vi "DB - [Config].[Controller].vi"(4 "[SystemId]":string="SRSB-A1", 6 "[PlantId]":string="4070", 7 "DB Connection":T2={"Open"=TRUE, "Close"=TRUE}, 8 "error in (no error)":errorcluster, 9 "DB.Schema.Table \nSRTRS.Config.Controller":string="SRTRS.Config.Controller", 10 "DB.Schema.Table\nSRTRS.Config.SysControlRelation":string="SRTRS.Config.SysControlRelation", 11 "connection reference":T1) -> (0 "SUMMARY":errorcluster, 2 "data":string[](array[string]), 3 "connection reference":T1)   [LabVIEW 2013]
uses:
  <vilib>/addons/database/Connection.llb/Conn ObjectReference.ctl
  Controls/DB - OpenClose.ctl
  <vilib>/addons/database/Connection.llb/Conn Execute.vi
  <vilib>/addons/database/Recordset.llb/Rec Fetch Recordset Data (R).vi
  <vilib>/addons/database/Recordset.llb/Rec Destroy - Connection.vi
  Controls/Global SRTRS.vi
  <vilib>/addons/database/Connection.llb/DB Tools Open Connec (String).vi
  <vilib>/addons/database/_DB Variant To Data/Database Variant To Data.xnode
  <vilib>/addons/database/NI_Database_API.lvlib
panel:
  out "Close":errorcluster
  in  "DB.Schema.Table \nNA":string
  out "SQL Statement":string
  out "Connection Information":T3={"Connection "="SQL Server 32bit HPEnvy", "Username"="admin", "Password"="admin123"}
  # "2014-10-27 14:11\n[IpAddress]                                                              [ChannelMapping]"
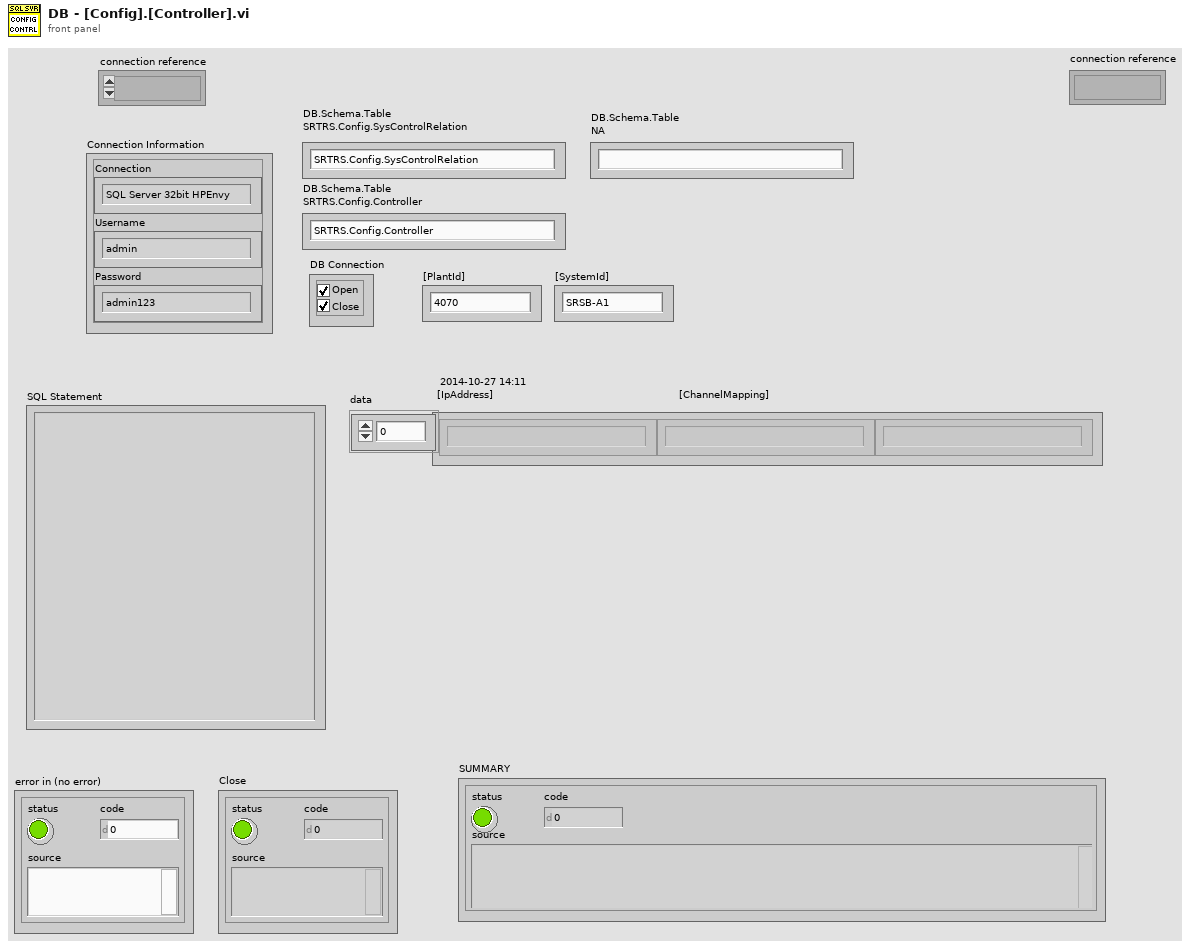
[diagram p1: front panel]
types:
  T1 = typedef "NI_Database_API.lvlib/Conn ObjectReference.ctl" = refnum<k1>
  T2 = typedef "DB - OpenClose.ctl" = cluster{"Open":bool, "Close":bool}
  T3 = cluster{"Connection ":string, "Username":string, "Password":string}
  T4 = typedef "Enum - InteractiveMode-SubVIMode.ctl" = enum16{"Interactive", "subVI Mode"}
  T5 = typedef "DB - DB.Schema.Table.ctl" = cluster{"DB":string, "Schema":string, "Table":string}
  T6 = typedef "Connection Information Cluster.ctl" = cluster{"Connection ":string, "Username":string, "Password":string}
  T7 = typedef "NI_Database_API.lvlib/Rec ObjectReference.ctl" = refnum<k1>
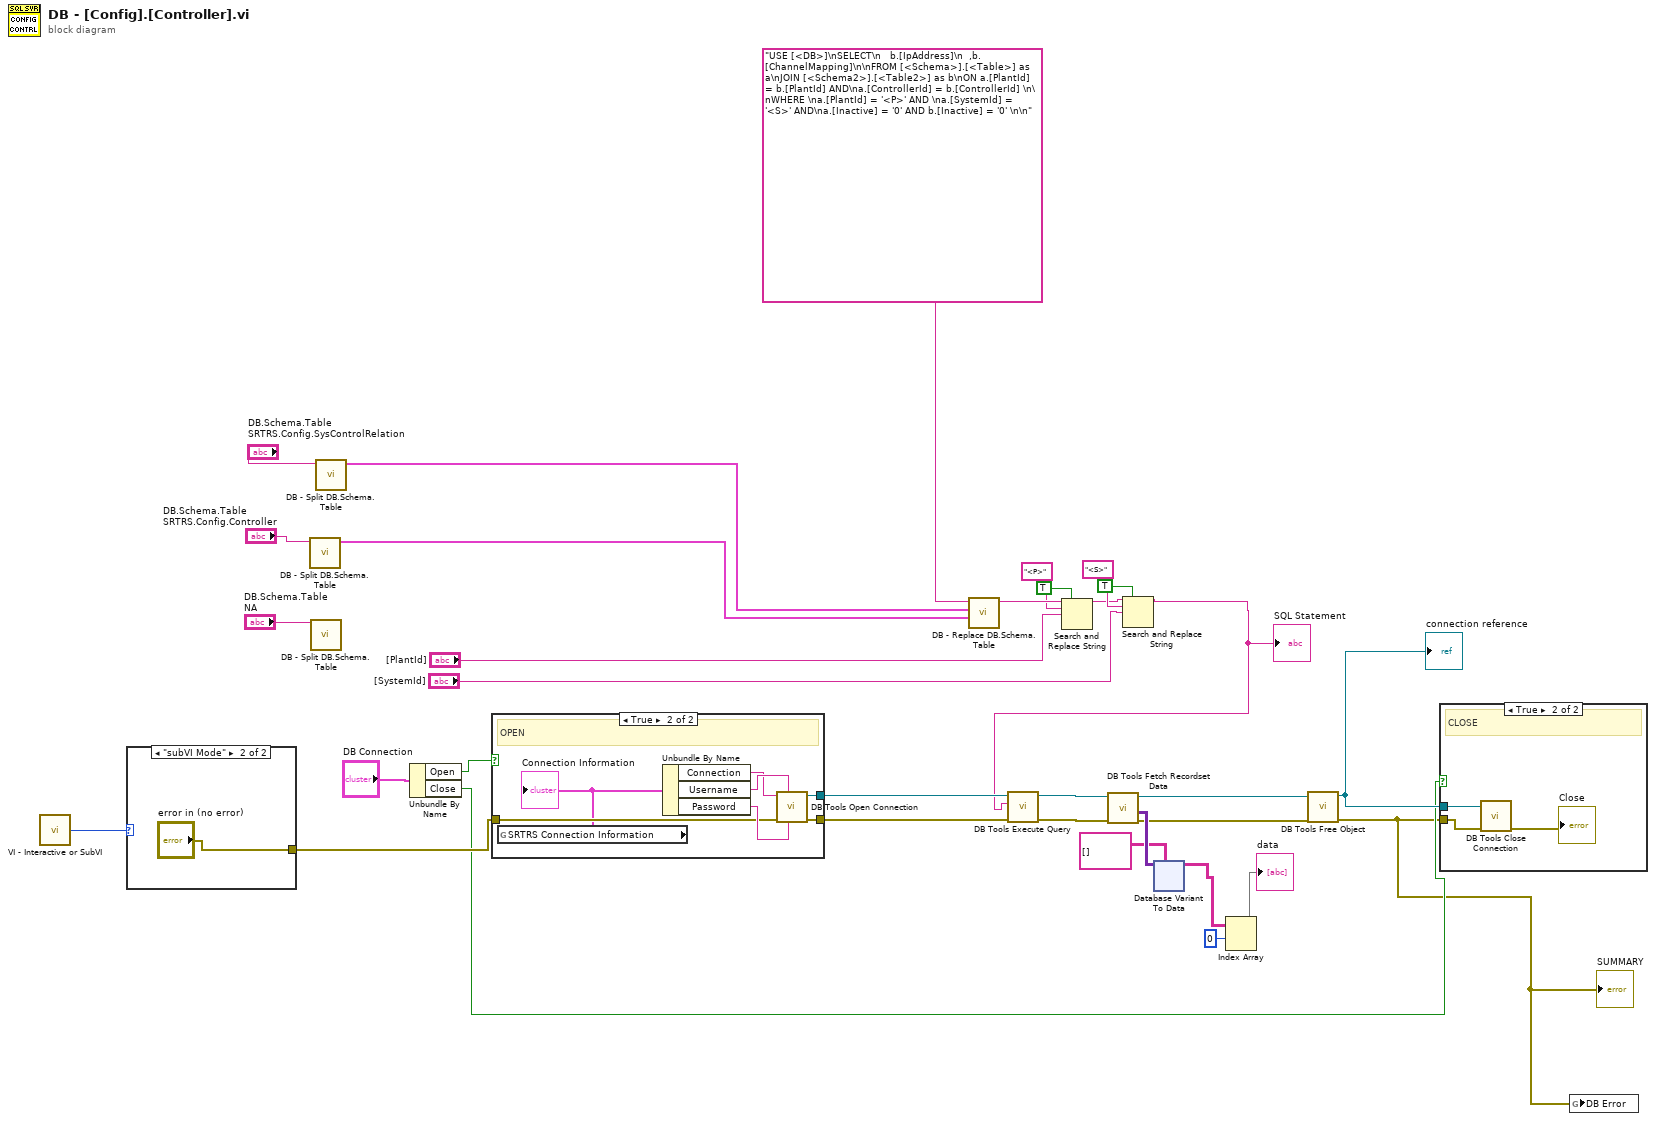
[diagram p0: block diagram]
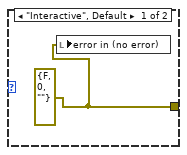
[diagram p3: hidden frame]
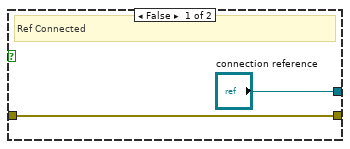
[diagram p4: hidden frame]
diagram:
  n1 = call "VI - Interactive or SubVI.vi"() -> ("Mode"=w31:T4)  [unwired: 5 in]
  n2 = case shown="\"subVI Mode\"" w31 {
    tunnel: [w34 "error in (no error)"] -> w30
    frame "Interactive", Default {
      w34 = errorcluster {"status"=FALSE, "code"=0, "source"=""} ("error in (no error)")
      n3 = local write "error in (no error)"(w34) -> ()
    }
    frame "subVI Mode" {
    }
  }
  n4 = call "DB - Split DB.Schema.Table.vi"("DB.Schema.Table"="DB.Schema.Table \nSRTRS.Config.Controller") -> ("DB.Schema.Table"=w12:T5)  [unwired: 10 in]
  n5 = call "DB - Split DB.Schema.Table.vi"("DB.Schema.Table"="DB.Schema.Table \nNA") -> ()  [unwired: 10 in, 1 out]
  n6 = call "DB - Split DB.Schema.Table.vi"("DB.Schema.Table"="DB.Schema.Table\nSRTRS.Config.SysControlRelation") -> ("DB.Schema.Table"=w17:T5)  [unwired: 10 in]
  n7 = Unbundle By Name("DB Connection") -> ("Open"=w32:bool, "Close"=w20:bool)
  n8 = case shown="True" w32 {
    tunnel: ["connection reference" w41] -> w23
    tunnel: w30 -> [w36 w40]
    tunnel: [w36 w39] -> w22
    frame False {
      # "Ref Connected"
    }
    frame True {
      # "OPEN"
      n9 = global read "Global SRTRS.vi" "SRTRS Connection Information"() -> (w38:T6)
      "Connection Information" <- w38
      n10 = Unbundle By Name(w38) -> ("Connection"=w43:string, "Username"=w44:string, "Password"=w42:string)
      n11 = call-poly <vilib>:"DB Tools Open Connection.vi"("password"=w42, "userID"=w44, "error in (no error)"=w40, "connection information"=w43) -> ("error out"=w39:errorcluster, "connection reference"=w41:T1)  [unwired: 4 in]
    }
  }
  n12 = call "DB - Replace DB.Schema.Table.vi"("DB.Schema.Table 2"=w12, "DB.Schema.Table"=w17, "string in"="USE [<DB>]\nSELECT\n   b.[IpAddress]\n  ,b.[ChannelMapping]\n\nFROM [<Schema>].[<Table>] as a\nJOIN [<Schema2>].[<Table2>] as b\nON a.[PlantId] = b.[PlantId] AND\na.[ControllerId] = b.[ControllerId] \n\nWHERE \na.[PlantId] = '<P>' AND \na.[SystemId] = '<S>' AND\na.[Inactive] = '0' AND b.[Inactive] = '0' \n\n") -> ("string out"=w15:string)  [unwired: 7 in, 1 out]
  n13 = Search and Replace String(replace all?=TRUE ("replace all? (F)"), input string=w15, search string="<P>", replace string="[PlantId]") -> (result string=w6:string)  [unwired: 4 in, 3 out]
  n14 = Search and Replace String(replace all?=TRUE ("replace all? (F)"), input string=w6, search string="<S>", replace string="[SystemId]") -> (result string=w4:string)  [unwired: 4 in, 3 out]
  "SQL Statement" <- w4
  n15 = call-poly <vilib>:"DB Tools Execute Query.vi"("error in (no error)"=w22, "SQL query"=w4, "connection reference"=w23) -> ("error out"=w29:errorcluster, "recordset reference"=w28:T7)  [unwired: 5 in]
  n16 = call-poly <vilib>:"DB Tools Fetch Recordset Data.vi"("error in (no error)"=w29, "recordset reference"=w28) -> ("error out"=w24:errorcluster, "recordset data"=w27:variant[][], "recordset reference out"=w25:T7)  [unwired: 3 in]
  n17 = xnode "Database Variant To Data"("database variant"=w27, "type"=string[][] []) -> ("data"=w3:string[][])  [unwired: 1 in, 1 out]
  n18 = Index Array(array=w3, index (row)=0) -> (element=→"data":string[])  [unwired: 1 in]
  n19 = call-poly <vilib>:"DB Tools Free Object.vi"("error in (no error)"=w24, "recordset reference"=w25) -> ("error out"=w10:errorcluster, "connection reference"=w21:T1)  [unwired: 8 in]
  "SUMMARY" <- w10
  "connection reference" <- w21
  n20 = case shown="True" w20 {
    tunnel: w21 -> [_ w47]
    tunnel: w10 -> [_ w46]
    frame False {
      # "Ref Connected"
    }
    frame True {
      # "CLOSE"
      n21 = call <vilib>:"DB Tools Close Connection.vi"("error in (no error)"=w46, "connection reference"=w47) -> ("error out"=→"Close":errorcluster)  [unwired: 5 in]
    }
  }
  n22 = global write "Global SRTRS.vi" "DB Error"(w10) -> ()
